vi "Integrieren.vi"(1 "Integrieren1":bool, 2 "Integral1":dbl, 4 "Integrieren2":bool, 5 "Integral2":dbl, 6 "Int.Start1":dbl, 8 "Int.Stop1":dbl, 10 "Int.Start2":dbl, 11 "HorstProbenflußNr.":i32, 12 "Int.Stop2":dbl) -> (15 "Integrieren1":bool, 16 "Integral1":dbl, 18 "Integrieren2":bool, 19 "Integral2":dbl)   [LabVIEW 2017]
uses:
  GVZeitenZyklen.vi
  GVProbenvol.vi
  GVMWHorst.vi
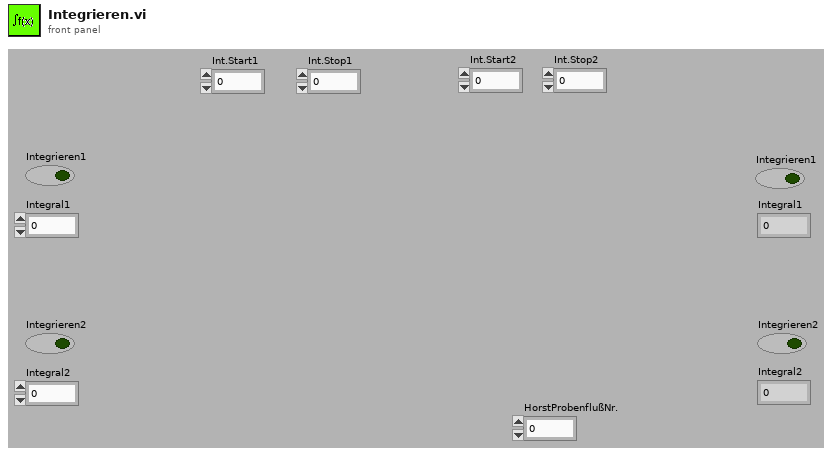
[diagram p1: front panel]
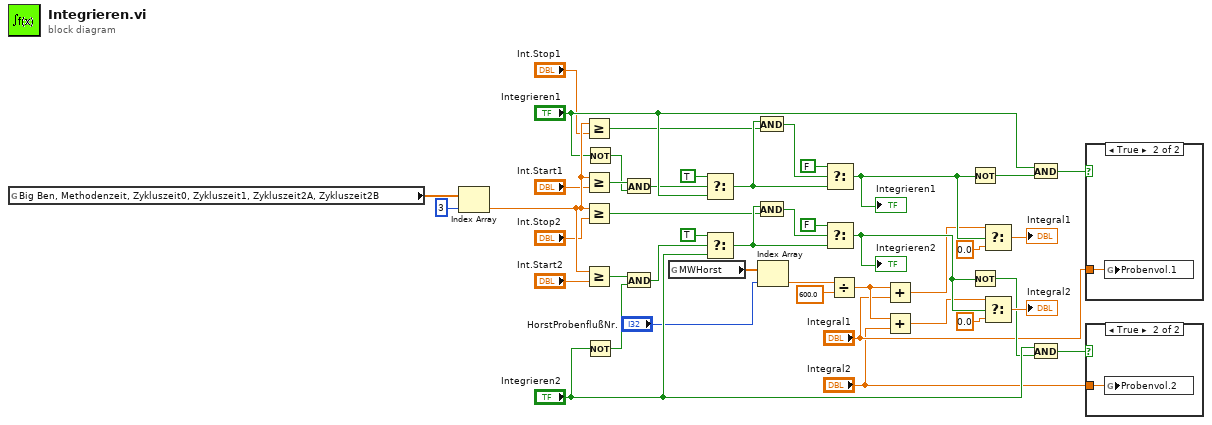
[diagram p0: block diagram]
diagram:
  n1 = global read "GVZeitenZyklen.vi" "Big Ben, Methodenzeit, Zykluszeit0, Zykluszeit1, Zykluszeit2A, Zykluszeit2B"() -> (w2:dbl[])
  n2 = Index Array(array=w2, index=3 ("Index")) -> (element=w40:dbl)
  n3 = Greater Or Equal?(x=w40, y="Int.Stop1") -> (x >= y?=w16:bool)
  n4 = Greater Or Equal?(x=w40, y="Int.Start1") -> (x >= y?=w13:bool)
  n5 = Greater Or Equal?(x=w40, y="Int.Stop2") -> (x >= y?=w32:bool)
  n6 = Greater Or Equal?(x=w40, y="Int.Start2") -> (x >= y?=w29:bool)
  n7 = Not(x="Integrieren1") -> (.not. x?=w12:bool)
  n8 = Not(x="Integrieren2") -> (.not. x?=w28:bool)
  n9 = And(x=w13, y=w12) -> (x .and. y?=w14:bool)
  n10 = And(x=w29, y=w28) -> (x .and. y?=w30:bool)
  n11 = global read "GVMWHorst.vi" "MWHorst"() -> (w1:dbl[])
  n12 = Select(t=TRUE, s=w14, f="Integrieren1") -> (s? t:f=w20:bool)
  n13 = Select(t=TRUE, s=w30, f="Integrieren2") -> (s? t:f=w36:bool)
  n14 = And(x=w20, y=w16) -> (x .and. y?=w17:bool)
  n15 = And(x=w36, y=w32) -> (x .and. y?=w33:bool)
  n16 = Index Array(array=w1, index="HorstProbenflußNr.") -> (element=w8:dbl)
  n17 = Select(t=FALSE, s=w17, f=w20) -> (s? t:f=w25:bool)
  "Integrieren1" <- w25
  n18 = Select(t=FALSE, s=w33, f=w36) -> (s? t:f=w44:bool)
  "Integrieren2" <- w44
  n19 = Divide(x=w8, y=600.0) -> (x/y=w41:dbl)
  n20 = Add(x=w41, y="Integral1") -> (x+y=w21:dbl)
  n21 = Add(x=w41, y="Integral2") -> (x+y=w37:dbl)
  n22 = Not(x=w25) -> (.not. x?=w26:bool)
  n23 = Not(x=w44) -> (.not. x?=w39:bool)
  n24 = Select(t=w21, s=w25, f=0.0) -> (s? t:f=→"Integral1":dbl)
  n25 = Select(t=w37, s=w44, f=0.0) -> (s? t:f=→"Integral2":dbl)
  n26 = And(x="Integrieren1", y=w26) -> (x .and. y?=w6:bool)
  n27 = And(x="Integrieren2", y=w39) -> (x .and. y?=w4:bool)
  n28 = case shown="True" w6 {
    tunnel: "Integral1" -> [_ w45]
    frame False {
    }
    frame True {
      n29 = global write "GVProbenvol.vi" "Probenvol.1"(w45) -> ()
    }
  }
  n30 = case shown="True" w4 {
    tunnel: "Integral2" -> [_ w46]
    frame False {
    }
    frame True {
      n31 = global write "GVProbenvol.vi" "Probenvol.2"(w46) -> ()
    }
  }
